vi "Volts_to_temperature_(SubVI).vi"(4 "ch_data_string":string, 7 "error in":errorcluster, 16 "koeff. cluster":T1) -> (20 "T solvation":dbl, 21 "meas_voltage":dbl, 27 "error out":errorcluster)   [LabVIEW 2015]
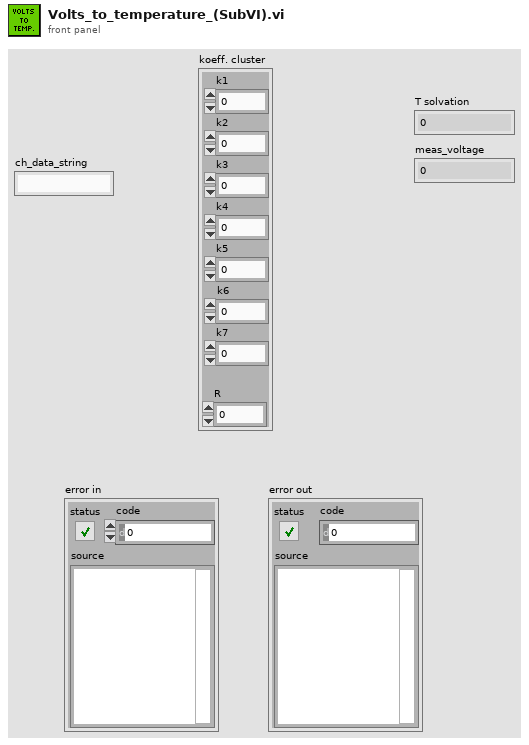
[diagram p1: front panel]
types:
  T1 = cluster{"k1":ext, "k2":ext, "k3":ext, "k4":ext, "k5":ext, "k6":ext, "k7":ext, "R":ext}
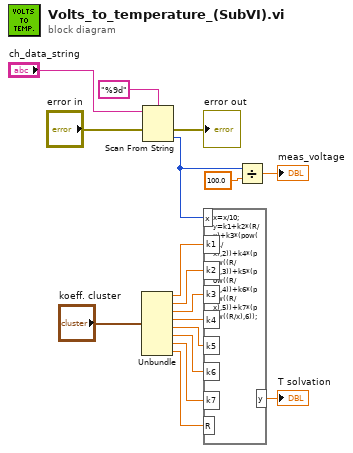
[diagram p0: block diagram]
diagram:
  n1 = Unbundle("koeff. cluster") -> ("k1"=w8:ext, "k2"=w6:ext, "k3"=w5:ext, "k4"=w4:ext, "k5"=w3:ext, "k6"=w2:ext, "k7"=w1:ext, "R"=w7:ext)
  n2 = Scan From String(format string="%9d", input string="ch_data_string", error in="error in") -> (error out=→"error out":errorcluster, output 1=w13:i32)  [unwired: 2 in, 2 out]
  n3 = formula code="x=x/10;\ny=k1+k2*(R/x)+k3*(pow((R/x),2))+k4*(pow((R/x),3))+k5*(pow((R/x),4))+k6*(pow((R/x),5))+k7*(pow((R/x),6));"("x"=w13, "k1"=w8, "k2"=w6, "k3"=w5, "k4"=w4, "k5"=w3, "k6"=w2, "k7"=w1, "R"=w7) -> ("y"=→"T solvation":dbl)
  n4 = Divide(x=w13, y=100.0) -> (x/y=→"meas_voltage":dbl)
